vi "StorePosition.vi"(8 "error in (no error)":errorcluster, 9 "Units":T1, 10 "Name":string, 11 "XYStage":refnum<class "XYStage.lvclass">) -> (0 "error out":errorcluster, 3 "XYStage out":refnum<class "XYStage.lvclass">)   [LabVIEW 2013, in "XYStage.lvclass"]
doc: "---------------------------------------------------------------\nJKI State Machine Objects™\nhttp://jki.net/state-machine-objects/\nCopyright (C) 2005-2015, JKI <info@jki.net>\nALL RIGHTS RESERVEDJKI State Machine Objects (SMO) 1.0.0.4\nJKI - JKI\nCopyright (c) 2015, JKI"
uses:
  XYStage.lvclass
  Typedefs/(real)Coords--Cluster.ctl
  utilities/SMO.Dictionary/SMO.Dictionary.lvclass
panel:
  # "For instructions on how to use the JKI State Machine Objects, examples and video tutorials, visit:\nhttp://jki.net/state-machine-objects/\n\nJKI State Machine Objects™\nhttp://jki.net/state-machine-objects/\nCopyright (C) 2005-2015, JKI <info@jki.net>\nALL RIGHTS RESERVED"
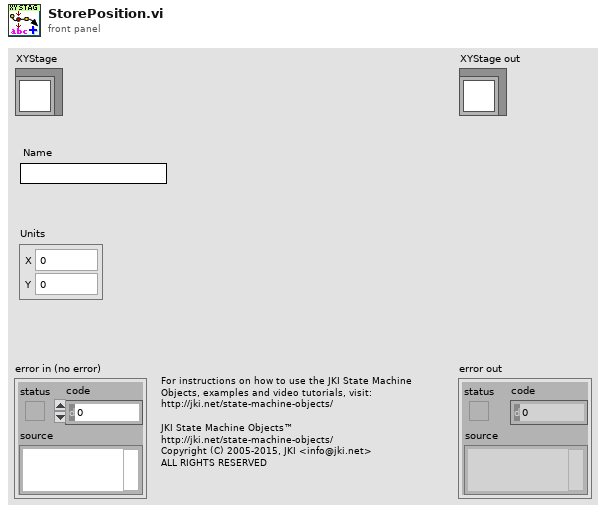
[diagram p1: front panel]
types:
  T1 = typedef "XYStage.lvclass/(real)Coords--Cluster.ctl" = cluster{"X":dbl, "Y":dbl}
  T2 = typedef "XYStage.lvclass/Dependencies--Cluster.ctl" = cluster{"Positions":refnum<class "SMO.Dictionary.Variant.lvclass">}
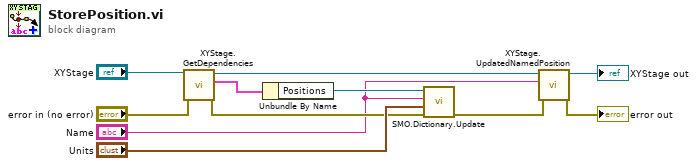
[diagram p0: block diagram]
diagram:
  n1 = call "XYStage.GetDependencies.vi"("error in (no error)"="error in (no error)", "XYStage"="XYStage") -> ("error out"=w6:errorcluster, "Dependencies"=w8:T2, "XYStage out"=w5:refnum<class "XYStage.lvclass">)  [unwired: 7 in]
  n2 = Unbundle By Name(w8) -> ("Positions"=w7:refnum<class "SMO.Dictionary.Variant.lvclass">)
  n3 = call "SMO.Dictionary.Update.vi"("error in (no error)"=w6, "Value"="Units", "Key (\"\": variant name)"="Name", "SMO.Dictionary"=w7) -> ("error out"=w2:errorcluster)  [unwired: 5 in, 2 out]
  n4 = call "XYStage.UpdatedNamedPosition.vi"("error in (no error)"=w2, "NewNamedPosition"="Name", "XYStage"=w5) -> ("error out"=→"error out":errorcluster, "XYStage out"=→"XYStage out":refnum<class "XYStage.lvclass">)  [unwired: 7 in]
